vi "Num Ref Set Value.vi"(8 "error in":errorcluster, 9 "Valid":bool, 10 "Value":variant, 11 "Num Ref":refnum<vi>) -> (0 "error out":errorcluster)   [LabVIEW 2018, in "Main Panel.lvlib" / "Main Panel.lvclass"]
uses:
  Main Panel.lvclass
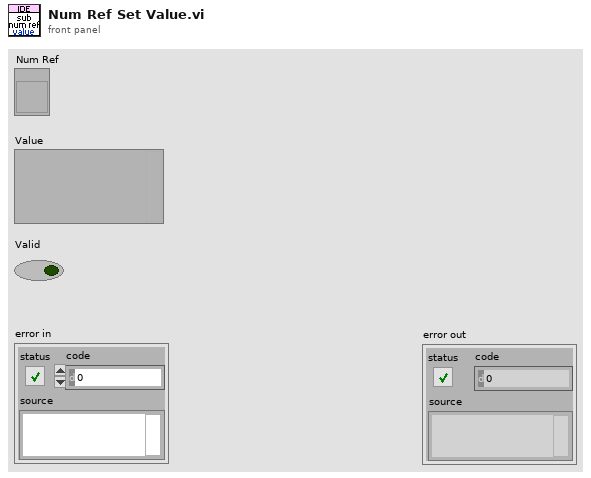
[diagram p1: front panel]
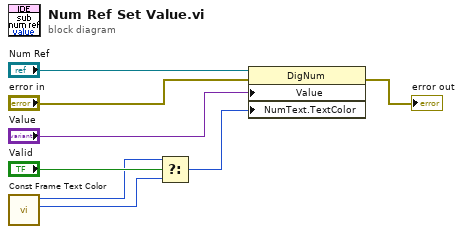
[diagram p0: block diagram]
diagram:
  n1 = call "Const Frame Text Color.vi"() -> ("invalid num color"=w1:u32, "valid num color"=w2:u32)  [unwired: 10 in]
  n2 = Select(t=w2, s="Valid", f=w1) -> (s? t:f=w3:u32)
  n3 = property class="DigNum"(reference="Num Ref", error in="error in", "Value"="Value", "NumText.TextColor"=w3) -> (error out=→"error out":errorcluster)  [unwired: 1 out]
